vi "Channel Read Write.vi"(11 "plugin gRPC address":string="localhost:51930") -> ()   [LabVIEW 2021, in "Template_Test_Helpers.lvlib"]
uses:
  Template_Test_Helpers.lvlib
  <vilib>/CIF Foundation/CIF Core/CIFCore/Common/Typedef/gRPC Reported Plugin Status.ctl
  <vilib>/CIF Foundation/CIF Core/CIFCore/Common/Typedef/Plugin State.ctl
  <vilib>/CIF Foundation/CIF Core/CIFCore/Common/Typedef/Timing Statistics.ctl
  <vilib>/CIF Foundation/CIF Core/CIFCore/Common/Typedef/Timing Stats Base.ctl
  <vilib>/CIF Foundation/CIF Core/CIFCore/Common/Typedef/FIFO Statistics.ctl
  <vilib>/CIF Foundation/CIF Core/CIFCore/Common/Typedef/Simple Error.ctl
  <vilib>/CIF Foundation/CIF Core/CIFCore/Common/Typedef/Monitor Doubles.ctl
  <vilib>/CIF Foundation/CIF Core/CIFCore/Common/Typedef/Monitor U64.ctl
  <vilib>/CIF Foundation/CIF Core/CIFCore/Common/Typedef/Monitor I64.ctl
  <vilib>/gRPC/LabVIEW gRPC Library/Client API/Close Client.vi
  <vilib>/CIF Foundation/CIF Core/CIFCore/Grpc/CIFCoreWrapper/CIFCoreWrapper.lvlib
  <vilib>/CIF Foundation/CIF Core/CIFCore/Class/CIFCorePlugin.lvclass
  Common/Typedef/Channels.ctl
  Common/Template_Common.lvlib
  Grpc/Template_wrapper/Template_Wrapper.lvlib
  <vilib>/CIF Foundation/CIF Core/CIFCore/Common/CIFCoreCommon.lvlib
panel:
  out "Node Status":T1 {"Monitor Doubles"."4" format="%#_9g"; "Monitor Doubles"."3" format="%#_9g"; "Monitor Doubles"."2" format="%#_9g"; "Monitor Doubles"."1" format="%#_9g"; "Timing Statistics (us)"."Period"."Avg" format="%_6g"}
  in  "EXIT":bool
  in  "Unload":bool
  out "Dbl out":dbl
  in  "U641":u64=45
  in  "Dbl2":dbl=3.0
  out "U64 out":u64
  out "error out":errorcluster
  in  "Dbl1":dbl=2.0
  # "Update plugin gRPC address including gRPC port and run on same target as the plugin code. \nExit will stop this VI.\nUnload will stop this VI and unload the plugin."
  # "Example Tag Read Write"
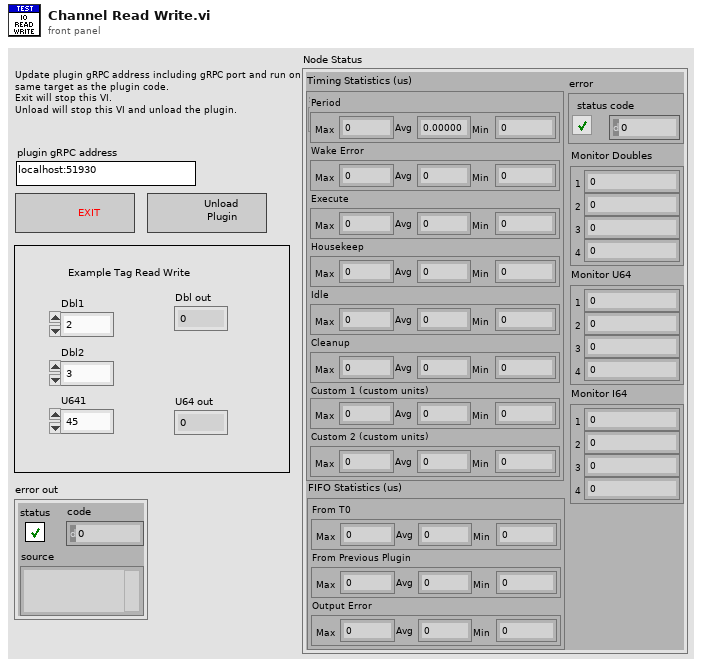
[diagram p1: front panel]
types:
  T1 = typedef "CIFCoreCommon.lvlib/gRPC Reported Plugin Status.ctl" = cluster{"State":T2, "Timing Statistics (us)":T3, "FIFO Statistics (us)":T5, "error":T6, "Monitor Doubles":T7, "Monitor U64":T8, "Monitor I64":T9}
  T2 = typedef "CIFCoreCommon.lvlib/Plugin State.ctl" = enum8{"Null", "Creating", "Listening", "Running", "CleaningUp", "Destroying", "Prepared", "FTE_Run"}
  T3 = typedef "CIFCoreCommon.lvlib/Timing Statistics.ctl" = cluster{"Period":T4, "Wake Error":T4, "Execute":T4, "Housekeep":T4, "Idle":T4, "Cleanup":T4, "Custom 1 (custom units)":T4, "Custom 2 (custom units)":T4}
  T4 = typedef "CIFCoreCommon.lvlib/Timing Stats Base.ctl" = cluster{"Max":i64, "Avg":dbl, "Min":i64}
  T5 = typedef "CIFCoreCommon.lvlib/FIFO Statistics.ctl" = cluster{"From T0":T4, "From Previous Plugin":T4, "Output Error":T4}
  T6 = typedef "CIFCoreCommon.lvlib/Simple Error.ctl" = cluster{"status":bool, "code":i32}
  T7 = typedef "CIFCoreCommon.lvlib/Monitor Doubles.ctl" = cluster{"1":dbl, "2":dbl, "3":dbl, "4":dbl}
  T8 = typedef "CIFCoreCommon.lvlib/Monitor U64.ctl" = cluster{"1":u64, "2":u64, "3":u64, "4":u64}
  T9 = typedef "CIFCoreCommon.lvlib/Monitor I64.ctl" = cluster{"1":i64, "2":i64, "3":i64, "4":i64}
  T10 = typedef "grpc-lvsupport-release.lvlib/grpcId.ctl" = u64
  T11 = typedef "CIFCoreChannel_client.lvlib/cif_management_common_Channel.ctl" = cluster{"name":string, "direction":T12, "type":string, "custom_config":u8[], "connected":bool, "connected_name":string, "forced":bool, "channel_pattern":T13}
  T12 = typedef "CIFCoreChannel_client.lvlib/cif_management_common_ChannelDirection.ctl" = enum32{"CHANNELDIRECTION_UNKNOWN", "CHANNELDIRECTION_PUBLISHER", "CHANNELDIRECTION_SUBSCRIBER"}
  T13 = typedef "CIFCoreChannel_client.lvlib/cif_management_common_ChannelPattern.ctl" = enum32{"CHANNELPATTERN_UNKNOWN", "CHANNELPATTERN_TAG", "CHANNELPATTERN_FIFO", "CHANNELPATTERN_MULTIFIFO", "CHANNELPATTERN_BACKPRESSUREFIFO"}
  T14 = typedef "Template_Common.lvlib/Channels.ctl" = enum16{"doubleout", "doublein1", "doublein2", "uint_out", "uint_in"}
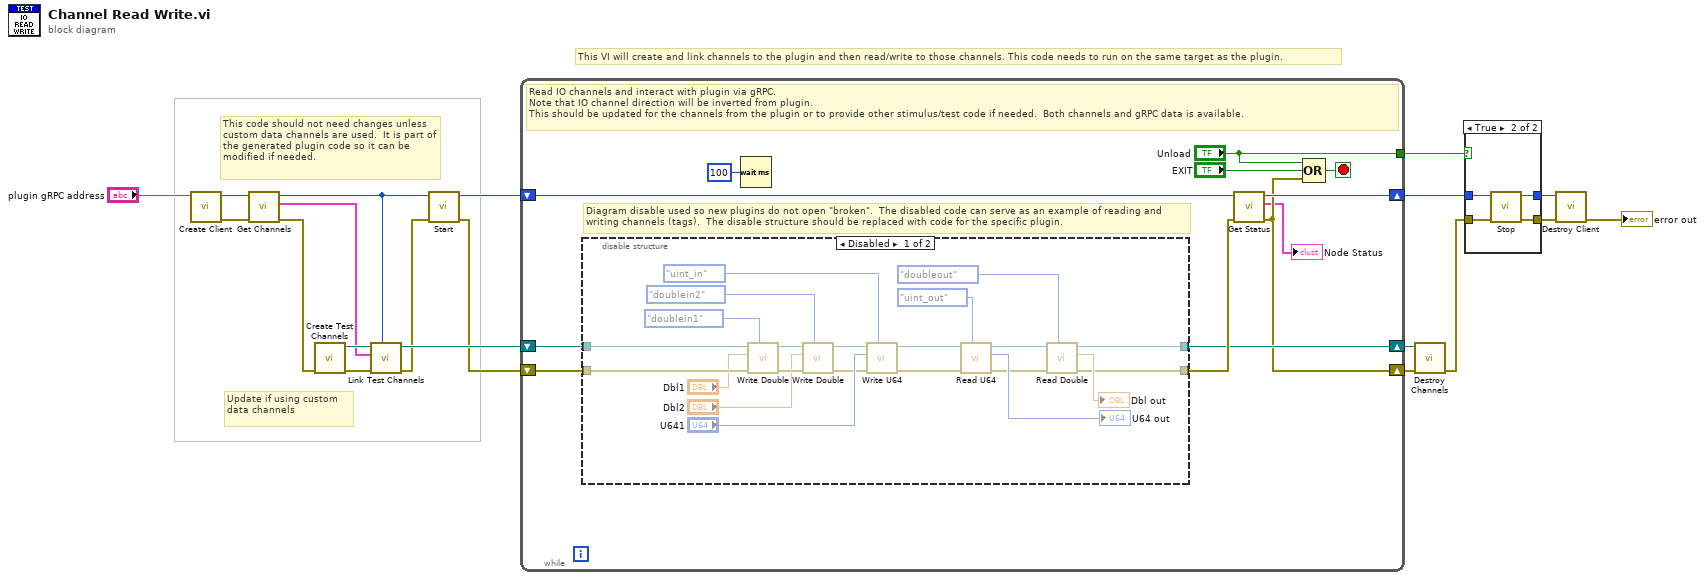
[diagram p0: block diagram]
diagram:
  # "Update if using custom data channels"
  # "This code should not need changes unless custom data channels are used.  It is part of the generated plugin code so it can be modified if needed."
  # "This VI will create and link channels to the plugin and then read/write to those channels. This code needs to run on the same target as the plugin."
  n1 = call "Create Client.vi"("address"="plugin gRPC address") -> ("error out"=w11:errorcluster, "gRPC ID Out"=w10:T10)  [unwired: 9 in]
  n2 = call <vilib>:"Get Channels.vi"("error in"=w11, "gRPC ID"=w10) -> ("error out"=w19:errorcluster, "Channels"=w15:T11[], "gRPC ID out"=w9:T10)  [unwired: 7 in]
  n3 = call "Create Test Channels.vi"("error in"=w19) -> ("error out"=w18:errorcluster, "CIFCorePlugin out"=w17:refnum<class "CIFCorePlugin.lvclass">)  [unwired: 9 in]
  n4 = call "Link Test Channels.vi"("gRPC ID in"=w9, "error in (no error)"=w18, "Channels"=w15, "CIFCorePlugin in"=w17) -> ("error out"=w7:errorcluster, "CIFCorePlugin out"=w16:refnum<class "CIFCorePlugin.lvclass">)  [unwired: 6 in]
  n5 = call <vilib>:"Start.vi"("error in"=w7, "gRPC ID"=w9) -> ("error out"=w6:errorcluster, "gRPC ID out"=w8:T10)  [unwired: 8 in]
  n6 = while {
    shift-right: [w26] -> w20
    shift-left: w16 -> [w32]
    shift-right: [w25] -> w14
    shift-left: w6 -> [w31]
    shift-right: [w29] -> w4
    shift-left: w8 -> [w30]
    tunnel: ["Unload"] -> w1
    stop <- w24 stop-if-true
    # "Diagram disable used so new plugins do not open \"broken\".  The disabled code can serve as an example of reading and writing channels (tags).  The disable structure should be replaced with code for the specific plugin."
    # "Read IO channels and interact with plugin via gRPC.\nNote that IO channel direction will be inverted from plugin.\nThis should be updated for the channels from the plugin or to provide other stimulus/test code if needed.  Both channels and gRPC data is available."
    n7 = disable-structure shown="Disabled" {
      disable-tunnel: w32 -> [w51 w56]
      disable-tunnel: w31 -> [w50 w55]
      disable-tunnel: [w36 w55] -> w27
      disable-tunnel: [w35 w56] -> w26
      frame Disabled {
        n8 = call <vilib>:"Write Double.vi"("Channel Index"=Channels."doublein1" ("Channels"), "error in (no error)"=w50, "Data"="Dbl1", "CIFCorePlugin in"=w51) -> ("error out"=w46:errorcluster, "CIFCorePlugin out"=w47:refnum<class "CIFCorePlugin.lvclass">)  [unwired: 6 in]
        n9 = call <vilib>:"Write Double.vi"("Channel Index"=Channels."doublein2" ("Channels"), "error in (no error)"=w46, "Data"="Dbl2", "CIFCorePlugin in"=w47) -> ("error out"=w42:errorcluster, "CIFCorePlugin out"=w41:refnum<class "CIFCorePlugin.lvclass">)  [unwired: 6 in]
        n10 = call <vilib>:"Write U64.vi"("Channel Index"=Channels."uint_in" ("Channels"), "error in (no error)"=w42, "Data"="U641", "CIFCorePlugin in"=w41) -> ("error out"=w33:errorcluster, "CIFCorePlugin out"=w34:refnum<class "CIFCorePlugin.lvclass">)  [unwired: 6 in]
        n11 = call <vilib>:"Read U64.vi"("Channel Index"=Channels."uint_out" ("Channels"), "error in (no error)"=w33, "CIFCorePlugin in"=w34) -> ("error out"=w39:errorcluster, "Data"=→"U64 out":u64, "CIFCorePlugin out"=w40:refnum<class "CIFCorePlugin.lvclass">)  [unwired: 6 in]
        n12 = call <vilib>:"Read Double.vi"("Channel Index"=Channels."doubleout" ("Channels"), "error in (no error)"=w39, "CIFCorePlugin in"=w40) -> ("error out"=w36:errorcluster, "Data"=→"Dbl out":dbl, "CIFCorePlugin out"=w35:refnum<class "CIFCorePlugin.lvclass">)  [unwired: 6 in]
      }
      frame Enabled {
      }
    }
    n13 = Wait (ms)(milliseconds to wait=u32 100) -> ()  [unwired: 1 out]
    n14 = call <vilib>:"Get Status.vi"("error in"=w27, "gRPC ID"=w30) -> ("error out"=w25:errorcluster, "Node Status"=→"Node Status":T1, "gRPC ID out"=w29:T10)  [unwired: 7 in]
    n15 = Compound Arithmetic op=OR("Unload", "EXIT", w25) -> (w24:bool)
  }
  n16 = call <vilib>:"Destroy Channels.vi"("error in (no error)"=w14, "CIFCorePlugin in"=w20) -> ("error out"=w5:errorcluster)  [unwired: 7 in, 2 out]
  n17 = case shown="True" w1 {
    tunnel: w5 -> [w57 w62]
    tunnel: w4 -> [w58 w61]
    tunnel: [w58 w60] -> w3
    tunnel: [w57 w59] -> w2
    frame False {
    }
    frame True {
      n18 = call <vilib>:"Stop.vi"("error in"=w62, "gRPC ID"=w61) -> ("error out"=w59:errorcluster, "gRPC ID out"=w60:T10)  [unwired: 8 in]
    }
  }
  n19 = call "Destroy Client.vi"("error in"=w2, "gRPC ID"=w3) -> ("error out"=→"error out":errorcluster)  [unwired: 9 in]
